vi "Read Abs_Waveform.lvclass.vi"(8 "error in (no error)":errorcluster, 11 "AbsFunc_Two Term_WFM in":refnum<class "AbsFunc_Two Term_WFM_Numeric.lvclass">) -> (0 "error out":errorcluster, 2 "Abs_Waveform.lvclass":refnum<class "Abs_Waveform.lvclass">, 3 "AbsFunc_Two Term_WFM out":refnum<class "AbsFunc_Two Term_WFM_Numeric.lvclass">)   [LabVIEW 2021, in "AbsFunc_Two Term_WFM_Numeric.lvclass"]
uses:
  AbsFunc_Two Term_WFM_Numeric.lvclass
  Abs_Types/Waveform/Abs_Waveform.lvclass
  AbsFunc_Two Term_WFM_Numeric.lvclass/AbsFunc_Two Term_WFM_Numeric.ctl
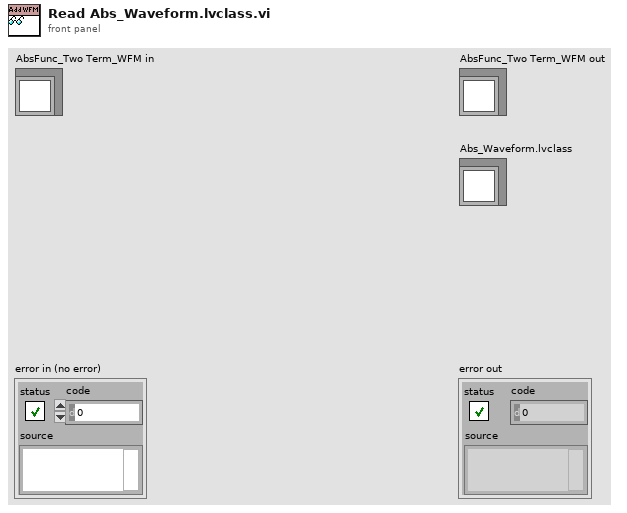
[diagram p1: front panel]
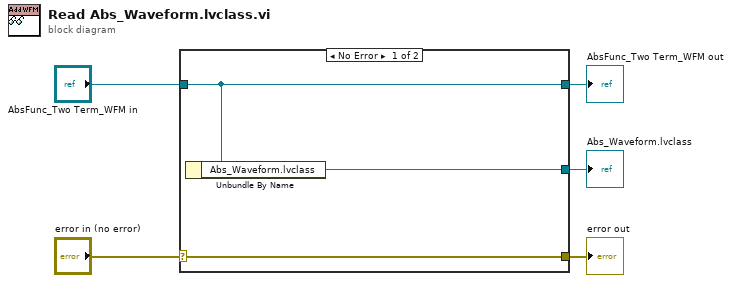
[diagram p0: block diagram]
diagram:
  n1 = case shown="No Error" "error in (no error)" {
    selector: "error in (no error)" -> [w8 w9]
    tunnel: [w8 w9] -> w4
    tunnel: [w7 w10] -> w2
    tunnel: "AbsFunc_Two Term_WFM in" -> [w7 w10]
    tunnel: [w6 _] -> w1
    frame No Error {
      n2 = Unbundle By Name(w7) -> ("Abs_Waveform.lvclass"=w6:refnum<class "Abs_Waveform.lvclass">)
    }
    frame Error {
    }
  }
  "error out" <- w4
  "AbsFunc_Two Term_WFM out" <- w2
  "Abs_Waveform.lvclass" <- w1
